vi "Move Cricket.vi"(8 "error in (no error)":errorcluster, 9 "Board Game in":refnum<class "Board Game.lvclass">, 10 "Packed refs":T1, 11 "Cricket in":refnum<class "Cricket.lvclass">) -> (0 "error out":errorcluster, 3 "Cricket out":refnum<class "Cricket.lvclass">)   [LabVIEW 2021, in "Cricket.lvclass"]
uses:
  Cricket.lvclass
  C:/Users/poche/Programs/LabVIEW/imposible snake/GameEl_class/GameEl.lvclass
  Board Game_class/Board Game.lvclass
  Application/Packed Refs.ctl
  GameEl_class/private/Enum Direction.ctl
  Cricket.lvclass/Cricket.ctl
  GameEl_class/GameEl.lvclass/GameEl.ctl
  Board Game_class/Board Game.lvclass/Board Game.ctl
  Snake_class/Snake.lvclass/Snake.ctl
  Imposible_Snake_v2/LVApp/Modules/Sound Manager/Typedefs/Sound Effects.ctl
  Board Game_class/Read Snake.vi
  Snake_class/Read Star.vi
  GameEl_class/Read position.vi
  Read Init Cricket.vi
  Snake_class/Snake.lvclass
  GameEl_class/GameEl.lvclass
  Imposible_Snake_v2/LVApp/Modules/Sound Manager/Sound Manager.lvlib
  Application/Game.lvclass
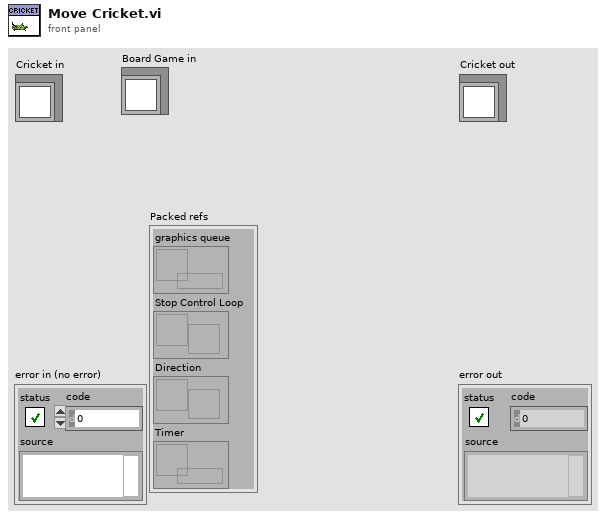
[diagram p1: front panel]
types:
  T1 = typedef "Game.lvclass/Packed Refs.ctl" = cluster{"graphics queue":refnum<queue>, "Stop Control Loop":refnum<user-event>, "Direction":refnum<notifier>, "Timer":refnum<data-value>}
  T2 = typedef "Sound Manager.lvlib/Sound Effects.ctl" = enum16{"Bomb In", "Bomb Out", "Bomb Touched", "Game Over", "Victory", "Eat", "10 Fruits", "Eat2", "Eat3", "Eat4", "MaxShield", "Shield", "10p", "Grape In", "Grape Out", "20p", "30p", "40p", "50p", "60p", "70p", "80p", "90p", "100p", "All shields cracked", "Mouse In", "Mouse Out", "Mouse Eaten", "Grape Eaten", "States Recover", "Broken Shield", "Bonus", "Happy Time", "explode", "Game over musica", "Back Music", "Shield Catch", "Evil lough", "Cricket In", "Cricket eaten", "Lets Go", "Jump1", "Jump2", "Jump3", "Unstoppable", "Troll Music", "winner", "menu"}
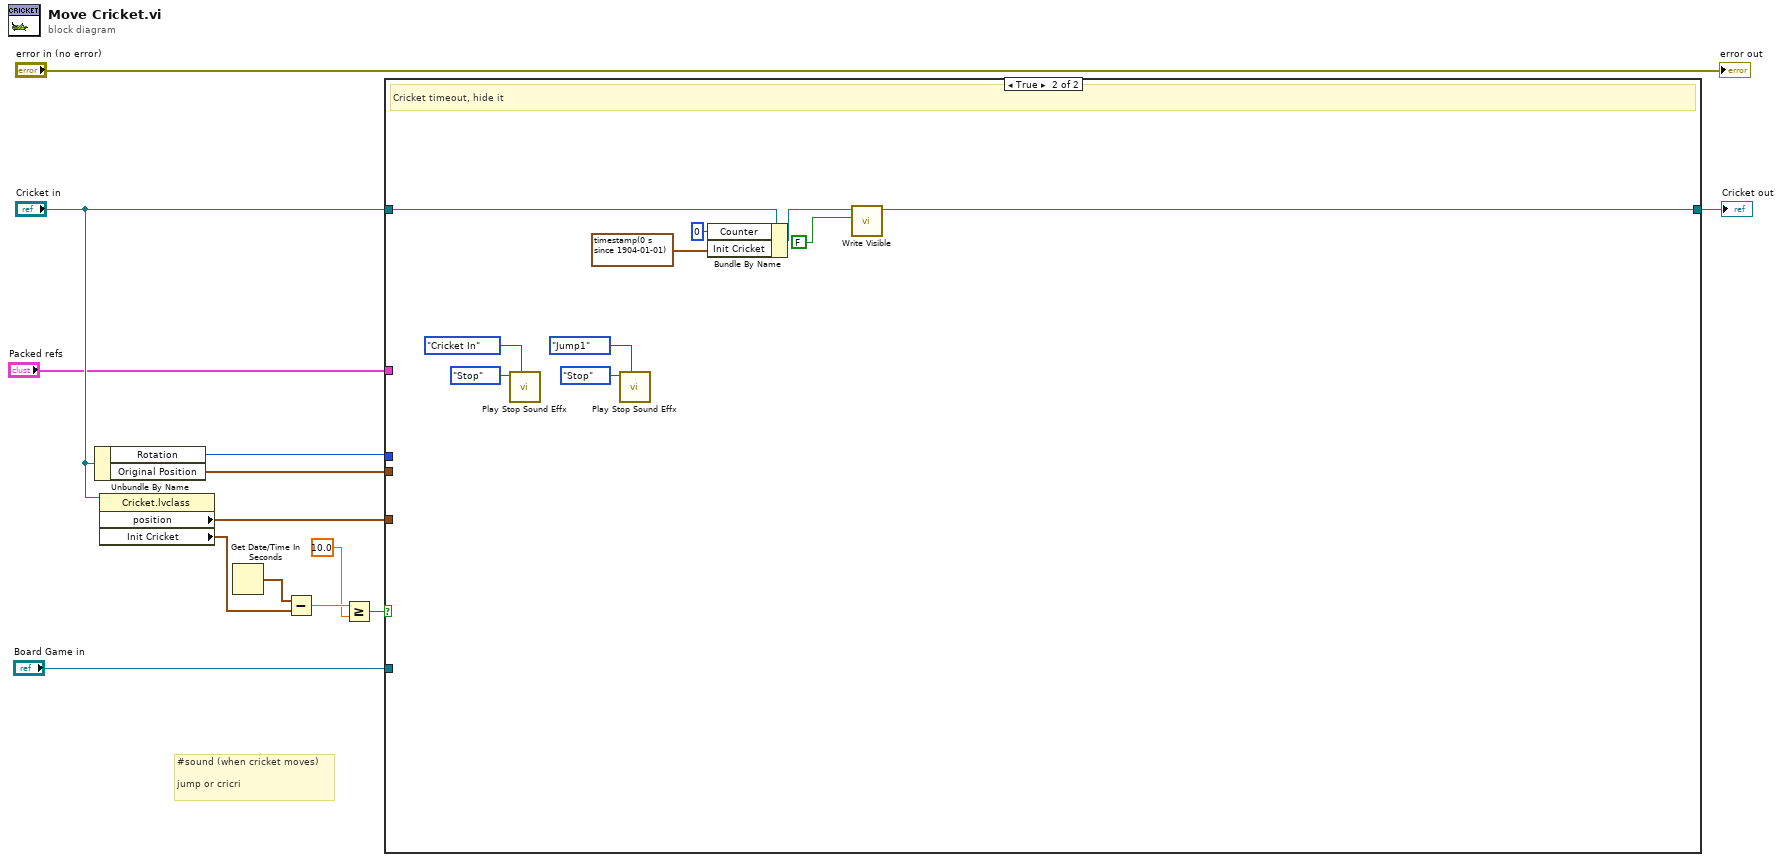
[diagram p0: block diagram]
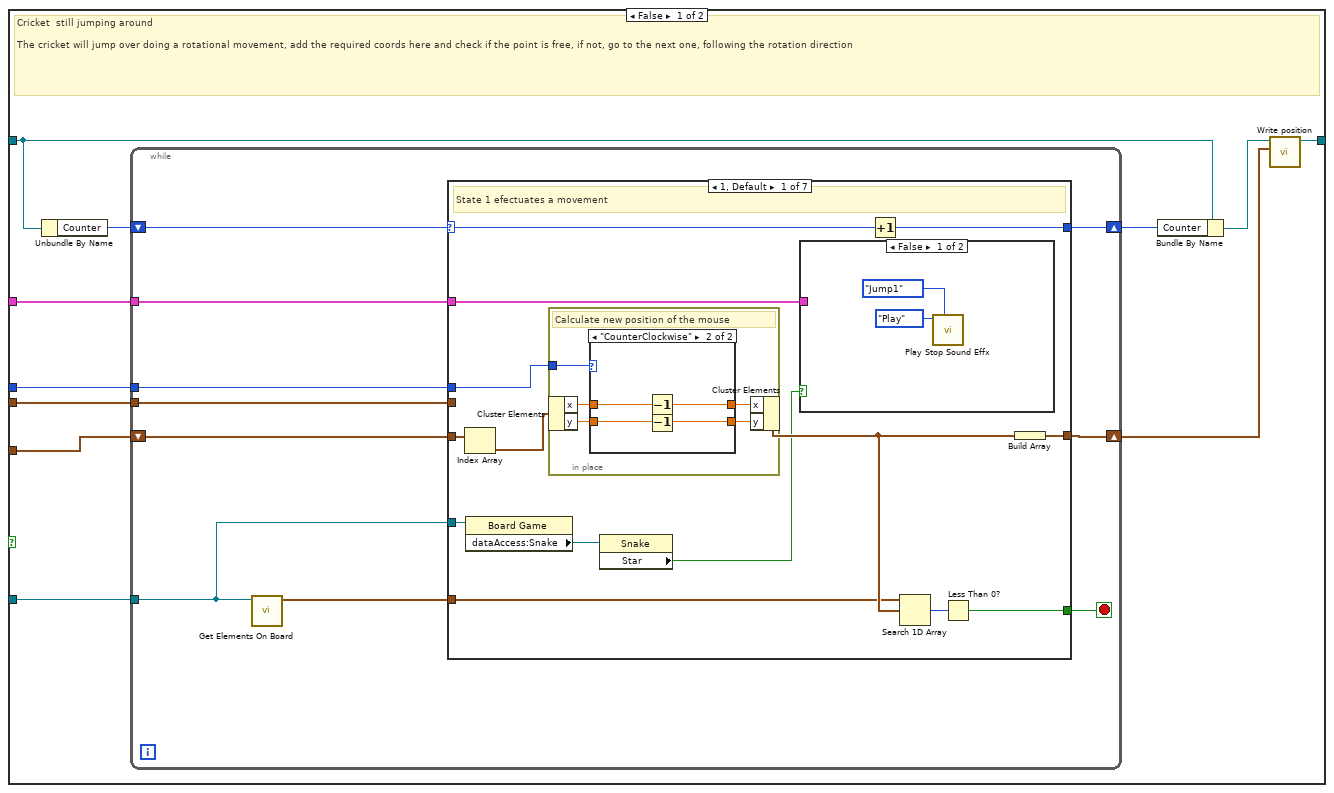
[diagram p2: hidden frame]
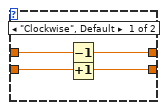
[diagram p4: hidden frame]
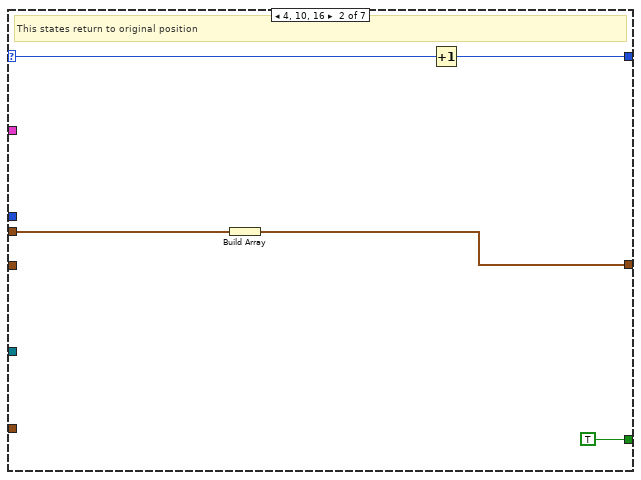
[diagram p5: hidden frame]
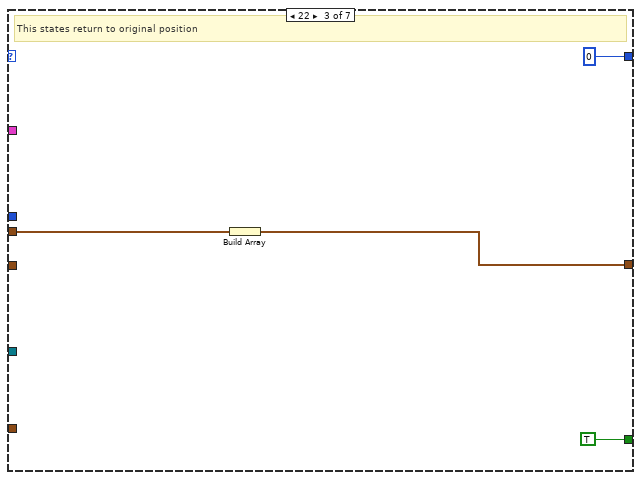
[diagram p6: hidden frame]
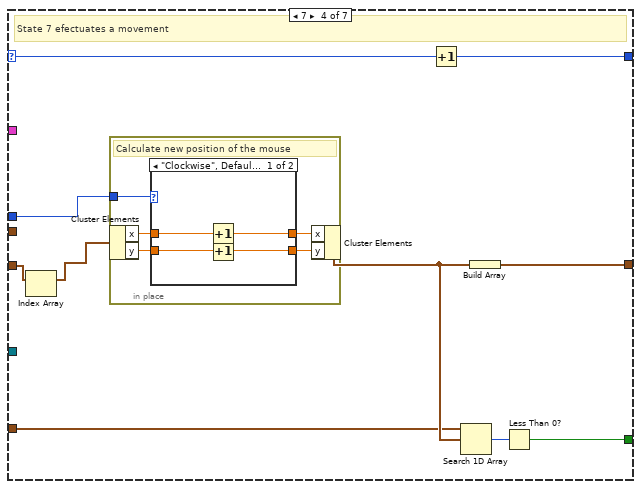
[diagram p7: hidden frame]
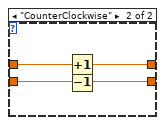
[diagram p8: hidden frame]
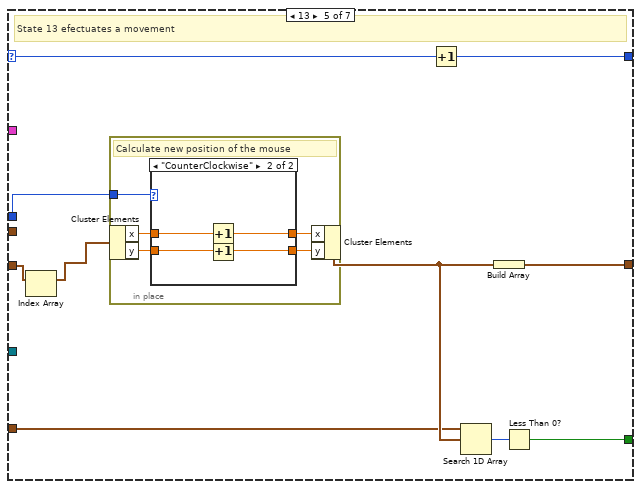
[diagram p9: hidden frame]
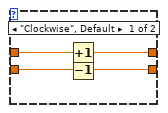
[diagram p10: hidden frame]
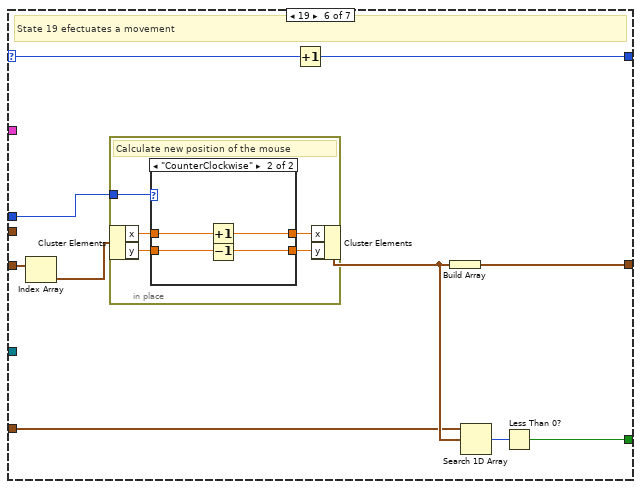
[diagram p11: hidden frame]
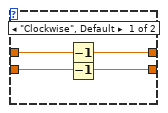
[diagram p12: hidden frame]
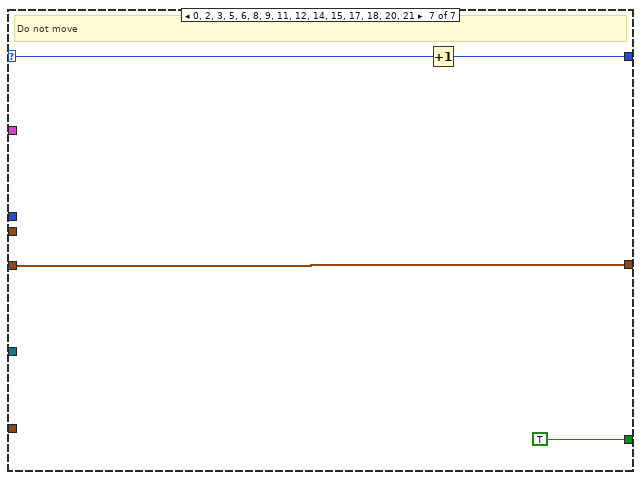
[diagram p13: hidden frame]
diagram:
  # "#sound (when cricket moves)\n\njump or cricri"
  n1 = Unbundle By Name("Cricket in") -> ("Rotation"=w12:enum16{"Clockwise", "CounterClockwise"}, "Original Position"=w2:cluster{"x":dbl, "y":dbl})
  n2 = property class="Cricket.lvclass"(reference="Cricket in") -> ("position"=w11:cluster{"x":dbl, "y":dbl}[], "Init Cricket"=w10:timestamp)  [unwired: 1 in, 2 out]
  n3 = Get Date/Time In Seconds() -> (seconds since 1Jan1904=w9:timestamp)
  n4 = Subtract(x=w9, y=w10) -> (x-y=w8:dbl)
  n5 = Greater Or Equal?(x=w8, y=10.0) -> (x >= y?=w4:bool)
  n6 = case shown="True" w4 {
    tunnel: w12 -> [w24 _]
    tunnel: "Cricket in" -> [w19 w152]
    tunnel: w11 -> [w23 _]
    tunnel: [w22 w150] -> w5
    tunnel: "Board Game in" -> [w20 _]
    tunnel: "Packed refs" -> [w14 _]
    tunnel: w2 -> [w15 _]
    frame False {
      # "Cricket  still jumping around\n\nThe cricket will jump over doing a rotational movement, add the required coords here and check if the point is free, if not, go to the next one, following the rotation direction"
      n7 = Unbundle By Name(w19) -> ("Counter"=w17:u32)
      n8 = while {
        tunnel: w24 -> [w34]
        tunnel: w20 -> [w25]
        shift-right: [w32] -> w21
        shift-left: w23 -> [w33]
        shift-right: [w30] -> w16
        shift-left: w17 -> [w31]
        tunnel: w15 -> [w27]
        tunnel: w14 -> [w26]
        stop <- w29 stop-if-true
        n9 = call "Get Elements On Board.vi"("Board Game in"=w25) -> ("position"=w28:cluster{"x":dbl, "y":dbl}[])  [unwired: 9 in, 1 out]
        n10 = case shown="1, Default" w31 {
          selector: w31 -> [w44 w68 _ w77 w100 w121 w145]
          tunnel: w34 -> [w38 _ _ w82 w105 w119 _]
          tunnel: w33 -> [w48 _ _ w81 w104 w128 w143]
          tunnel: [w45 w65 w71 w78 w101 w125 w143] -> w32
          tunnel: w28 -> [w40 _ _ w73 w96 w122 _]
          tunnel: [w43 w67 u32 0 ("Counter") w76 w99 w120 w144] -> w30
          tunnel: [w42 TRUE TRUE w75 w98 w124 TRUE] -> w29
          tunnel: w27 -> [_ w66 w72 _ _ _ _]
          tunnel: w26 -> [w39 _ _ _ _ _ _]
          tunnel: w25 -> [w37 _ _ _ _ _ _]
          frame 1, Default {
            # "State 1 efectuates a movement"
            n11 = Index Array(array=w48) -> (element=w47:cluster{"x":dbl, "y":dbl})  [unwired: 1 in]
            n12 = property class="Board Game"(reference=w37) -> ("dataAccess:Snake"=w36:refnum<class "Snake.lvclass">)  [unwired: 1 in, 2 out]
            n13 = in-place {
              in-place-border: w38 -> [w55]
              # "Calculate new position of the mouse"
              n14 = in-place-cluster #1(w47) -> ("x"=w54:dbl, "y"=w53:dbl)
              n15 = case shown="\"CounterClockwise\"" w55 {
                tunnel: w54 -> [w59 w63]
                tunnel: w53 -> [w58 w62]
                tunnel: [w57 w61] -> w51
                tunnel: [w56 w60] -> w52
                frame "Clockwise", Default {
                  n16 = Decrement(x=w59) -> (x-1=w57:dbl)
                  n17 = Increment(x=w58) -> (x+1=w56:dbl)
                }
                frame "CounterClockwise" {
                  n18 = Decrement(x=w63) -> (x-1=w61:dbl)
                  n19 = Decrement(x=w62) -> (x-1=w60:dbl)
                }
              }
              n20 = in-place-cluster #1("x"=w51, "y"=w52) -> (w46:cluster{"x":dbl, "y":dbl})
            }
            n21 = property class="Snake"(reference=w36) -> ("Star"=w35:bool)  [unwired: 1 in, 2 out]
            n22 = case shown="False" w35 {
              tunnel: w39 -> [_ _]
              frame False {
                n23 = call "Play Stop Sound Effx.vi"("Sound Effect"=Sound_Effects."Jump1", "Function"=enum16{"Play", "Stop"}."Play") -> ()  [unwired: 9 in, 1 out]
              }
              frame True {
              }
            }
            n24 = Increment(x=w44) -> (x+1=w43:u32)
            n25 = Search 1D Array(1D array=w40, element=w46) -> (index of element=w41:i32)  [unwired: 1 in]
            n26 = Less Than 0?(x=w41) -> (x < 0?=w42:bool)
            n27 = Build Array(w46) -> (w45:cluster{"x":dbl, "y":dbl}[])
          }
          frame 4, 10, 16 {
            # "This states return to original position"
            n28 = Build Array(w66) -> (w65:cluster{"x":dbl, "y":dbl}[])
            n29 = Increment(x=w68) -> (x+1=w67:u32)
          }
          frame 22 {
            # "This states return to original position"
            n30 = Build Array(w72) -> (w71:cluster{"x":dbl, "y":dbl}[])
          }
          frame 7 {
            # "State 7 efectuates a movement"
            n31 = Index Array(array=w81) -> (element=w80:cluster{"x":dbl, "y":dbl})  [unwired: 1 in]
            n32 = in-place {
              in-place-border: w82 -> [w87]
              # "Calculate new position of the mouse"
              n33 = in-place-cluster #2(w80) -> ("x"=w86:dbl, "y"=w85:dbl)
              n34 = case shown="\"Clockwise\", Default" w87 {
                tunnel: w86 -> [w91 w95]
                tunnel: w85 -> [w90 w94]
                tunnel: [w89 w93] -> w83
                tunnel: [w88 w92] -> w84
                frame "Clockwise", Default {
                  n35 = Increment(x=w91) -> (x+1=w89:dbl)
                  n36 = Increment(x=w90) -> (x+1=w88:dbl)
                }
                frame "CounterClockwise" {
                  n37 = Increment(x=w95) -> (x+1=w93:dbl)
                  n38 = Decrement(x=w94) -> (x-1=w92:dbl)
                }
              }
              n39 = in-place-cluster #2("x"=w83, "y"=w84) -> (w79:cluster{"x":dbl, "y":dbl})
            }
            n40 = Increment(x=w77) -> (x+1=w76:u32)
            n41 = Search 1D Array(1D array=w73, element=w79) -> (index of element=w74:i32)  [unwired: 1 in]
            n42 = Build Array(w79) -> (w78:cluster{"x":dbl, "y":dbl}[])
            n43 = Less Than 0?(x=w74) -> (x < 0?=w75:bool)
          }
          frame 13 {
            # "State 13 efectuates a movement"
            n44 = Index Array(array=w104) -> (element=w103:cluster{"x":dbl, "y":dbl})  [unwired: 1 in]
            n45 = in-place {
              in-place-border: w105 -> [w110]
              # "Calculate new position of the mouse"
              n46 = in-place-cluster #3(w103) -> ("x"=w109:dbl, "y"=w108:dbl)
              n47 = case shown="\"CounterClockwise\"" w110 {
                tunnel: w109 -> [w114 w118]
                tunnel: w108 -> [w113 w117]
                tunnel: [w112 w116] -> w106
                tunnel: [w111 w115] -> w107
                frame "Clockwise", Default {
                  n48 = Increment(x=w114) -> (x+1=w112:dbl)
                  n49 = Decrement(x=w113) -> (x-1=w111:dbl)
                }
                frame "CounterClockwise" {
                  n50 = Increment(x=w118) -> (x+1=w116:dbl)
                  n51 = Increment(x=w117) -> (x+1=w115:dbl)
                }
              }
              n52 = in-place-cluster #3("x"=w106, "y"=w107) -> (w102:cluster{"x":dbl, "y":dbl})
            }
            n53 = Increment(x=w100) -> (x+1=w99:u32)
            n54 = Search 1D Array(1D array=w96, element=w102) -> (index of element=w97:i32)  [unwired: 1 in]
            n55 = Build Array(w102) -> (w101:cluster{"x":dbl, "y":dbl}[])
            n56 = Less Than 0?(x=w97) -> (x < 0?=w98:bool)
          }
          frame 19 {
            # "State 19 efectuates a movement"
            n57 = Index Array(array=w128) -> (element=w127:cluster{"x":dbl, "y":dbl})  [unwired: 1 in]
            n58 = in-place {
              in-place-border: w119 -> [w133]
              # "Calculate new position of the mouse"
              n59 = in-place-cluster #4(w127) -> ("x"=w132:dbl, "y"=w131:dbl)
              n60 = case shown="\"CounterClockwise\"" w133 {
                tunnel: w132 -> [w137 w141]
                tunnel: w131 -> [w136 w140]
                tunnel: [w135 w139] -> w129
                tunnel: [w134 w138] -> w130
                frame "Clockwise", Default {
                  n61 = Decrement(x=w137) -> (x-1=w135:dbl)
                  n62 = Decrement(x=w136) -> (x-1=w134:dbl)
                }
                frame "CounterClockwise" {
                  n63 = Increment(x=w141) -> (x+1=w139:dbl)
                  n64 = Decrement(x=w140) -> (x-1=w138:dbl)
                }
              }
              n65 = in-place-cluster #4("x"=w129, "y"=w130) -> (w126:cluster{"x":dbl, "y":dbl})
            }
            n66 = Increment(x=w121) -> (x+1=w120:u32)
            n67 = Build Array(w126) -> (w125:cluster{"x":dbl, "y":dbl}[])
            n68 = Search 1D Array(1D array=w122, element=w126) -> (index of element=w123:i32)  [unwired: 1 in]
            n69 = Less Than 0?(x=w123) -> (x < 0?=w124:bool)
          }
          frame 0, 2, 3, 5, 6, 8, 9, 11, 12, 14, 15, 17, 18, 20, 21 {
            # "Do not move"
            n70 = Increment(x=w145) -> (x+1=w144:u32)
          }
        }
      }
      n71 = Bundle By Name(cluster=w19, "Counter"=w16) -> (w18:refnum<class "Cricket.lvclass">)
      n72 = call "Write position.vi"("position"=w21, "GameEl in"=w18) -> ("GameEl out"=w22:refnum<class "Cricket.lvclass">)  [unwired: 8 in, 1 out]
    }
    frame True {
      # "Cricket timeout, hide it"
      n73 = call "Play Stop Sound Effx.vi"("Sound Effect"=Sound_Effects."Cricket In", "Function"=enum16{"Play", "Stop"}."Stop") -> ()  [unwired: 9 in, 1 out]
      n74 = call "Play Stop Sound Effx.vi"("Sound Effect"=Sound_Effects."Jump1", "Function"=enum16{"Play", "Stop"}."Stop") -> ()  [unwired: 9 in, 1 out]
      n75 = Bundle By Name(cluster=w152, "Counter"=u32 0, "Init Cricket"=timestamp(0 s since 1904-01-01) ("Init Mouse")) -> (w151:refnum<class "Cricket.lvclass">)
      n76 = call "Write Visible.vi"("Visible"=FALSE, "GameEl in"=w151) -> ("GameEl out"=w150:refnum<class "Cricket.lvclass">)  [unwired: 8 in, 1 out]
    }
  }
  "Cricket out" <- w5
  "error out" <- "error in (no error)"
